vi "WaitForLimit.vi"(7 "Description":string, 8 "Command Info In":T1, 11 "Value":bool) -> (0 "Command Info Out":T1)   [LabVIEW 2018]
doc: "This template is useful for immediate subsystem actions that do not need deadband filtering\n\nBe sure to right-click and select New from Template and save with a new command name."
uses:
  <vilib>/Rock Robotics/WPI/Framework/Command Status Info.ctl
  <vilib>/Rock Robotics/WPI/Framework/Completion Status.ctl
  <vilib>/Rock Robotics/WPI/Framework/Completion Notifier.ctl
  Implementation/Hatch Intake Setpoints.ctl
  Implementation/Hatch Intake Operations.ctl
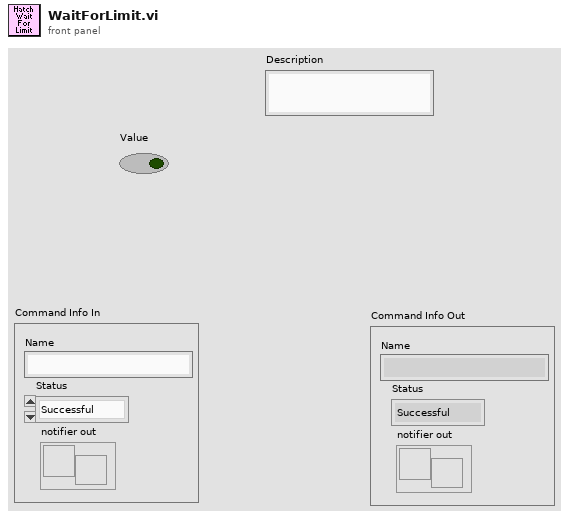
[diagram p1: front panel]
types:
  T1 = typedef "Command Status Info.ctl" = cluster{"Name":string, "Status":T2, "notifier out":T3}
  T2 = typedef "Completion Status.ctl" = enum16{"Successful", "Aborted", "Incomplete"}
  T3 = typedef "Completion Notifier.ctl" = refnum<notifier>
  T4 = typedef "Hatch Intake Setpoints.ctl" = cluster{"Operation":T5, "Collapsed?":bool, "Speed":dbl, "DistanceFromEnd":dbl}
  T5 = typedef "Hatch Intake Operations.ctl" = enum16{"Reserve", "Read Current", "SetValue", "WaitForLimit", "FloorHatchImmediate", "HatchAfterDriveAtDistance"}
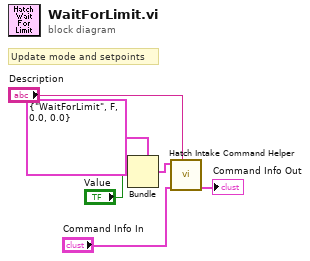
[diagram p0: block diagram]
diagram:
  # "Update mode and setpoints"
  n1 = Bundle(cluster=T4 {"Operation"=enum."WaitForLimit", "Collapsed?"=FALSE, "Speed"=0.0, "DistanceFromEnd"=0.0} ("SubSystem Data"), "Collapsed?"="Value") -> (w2:T4)  [unwired: 3 in]
  n2 = call "Hatch Intake Command Helper.vi"("Description"="Description", "Command Info In"="Command Info In", "SubSystem Data"=w2) -> ("Command Info Out"=→"Command Info Out":T1)  [unwired: 6 in, 2 out]
